vi "Get Signal.vi"(8 "Error in":errorcluster, 10 "Signal Name":string, 11 "CAN Frame in":refnum<class "CAN Frame.lvclass">) -> (0 "error out":errorcluster, 2 "Value":variant, 3 "CAN Frame out":refnum<class "CAN Frame.lvclass">)   [LabVIEW 2023, in "CAN Frame.lvclass"]
uses:
  CAN Frame.lvclass
  CAN Frame.lvclass/CAN Frame.ctl
  CAN Signal/CAN Signal.lvclass/CAN Signal.ctl
  CAN Signal/Get Start Bit.vi
  CAN Signal/Get Bit Length.vi
  CAN Signal/Get Data Type.vi
  CAN Signal/Get Scale.vi
  CAN Signal/Get Offset.vi
  CAN Signal/CAN Signal.lvclass
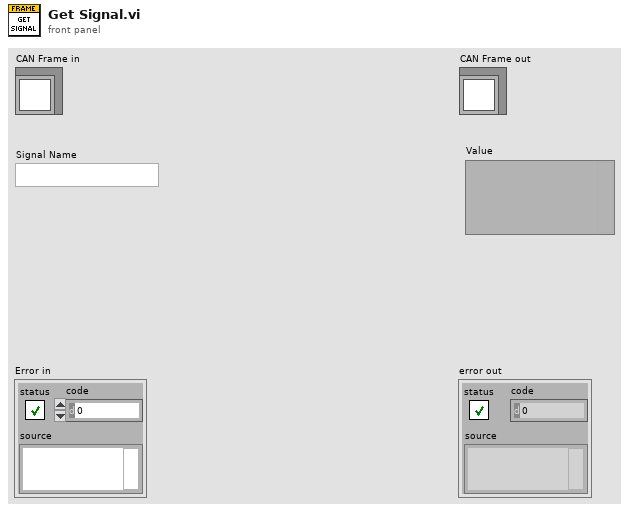
[diagram p1: front panel]
types:
  T1 = enum16{"Signed", "Unsigned", "IEEE Float", "Byte Array"}
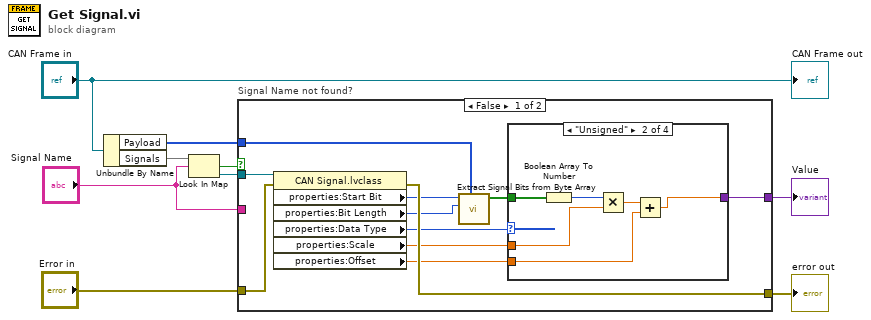
[diagram p0: block diagram]
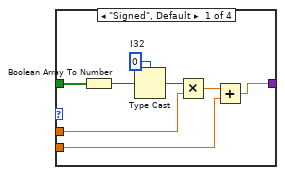
[diagram p2: hidden frame]
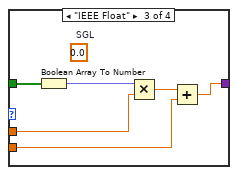
[diagram p3: hidden frame]
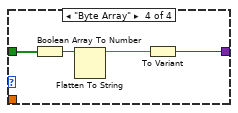
[diagram p4: hidden frame]
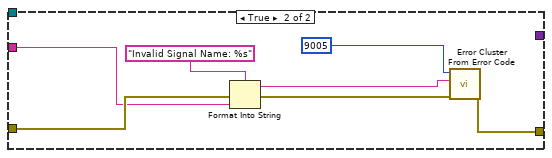
[diagram p5: hidden frame]
diagram:
  n1 = Unbundle By Name("CAN Frame in") -> ("Payload"=w2:u8[], "Signals"=w8:map{string, refnum<class "CAN Signal.lvclass">})
  n2 = Look In Map(map=w8, key="Signal Name") -> (key not found?=w5:bool, value=w6:refnum<class "CAN Signal.lvclass">)  [unwired: 1 in]
  n3 = case "Signal Name not found?" shown="False" w5 {
    tunnel: "Error in" -> [w20 w51]
    tunnel: w6 -> [w19 _]
    tunnel: "Signal Name" -> [_ w46]
    tunnel: [w18 w45] -> w3
    tunnel: w2 -> [w17 _]
    tunnel: [w13 _] -> w1
    frame False {
      n4 = property class="CAN Signal.lvclass"(reference=w19, error in=w20) -> (error out=w18:errorcluster, "properties:Start Bit"=w16:u32, "properties:Bit Length"=w15:u32, "properties:Data Type"=w14:T1, "properties:Scale"=w12:dbl, "properties:Offset"=w11:dbl)  [unwired: 1 out]
      n5 = call "Extract Signal Bits from Byte Array.vi"("Payload"=w17, "Bit Length"=w15, "Start Bit"=w16) -> ("Signal Bits"=w10:bool[])  [unwired: 8 in]
      n6 = case shown="\"Unsigned\"" w14 {
        tunnel: [w24 w31 w39 w43] -> w13
        tunnel: w12 -> [w25 w34 w40 _]
        tunnel: w11 -> [w23 w32 w38 _]
        tunnel: w10 -> [w21 w29 w37 w41]
        frame "Signed", Default {
          w27 = 0  # I32
          n7 = Boolean Array To Number(Boolean array=w21) -> (number=w22:u32)
          n8 = Type Cast(type=w27, x=w22) -> (*(type *) &x=w28:i32)
          n9 = Multiply(x=w28, y=w25) -> (x*y=w26:dbl)
          n10 = Add(x=w26, y=w23) -> (x+y=w24:dbl)
        }
        frame "Unsigned" {
          n11 = Boolean Array To Number(Boolean array=w29) -> (number=w30:u32)
          n12 = Multiply(x=w30, y=w34) -> (x*y=w33:dbl)
          n13 = Add(x=w33, y=w32) -> (x+y=w31:dbl)
        }
        frame "IEEE Float" {
          (unwired) sgl 0.0  # SGL
          n14 = Boolean Array To Number(Boolean array=w37) -> (number=w35:fxp<+/-,32,16>)
          n15 = Multiply(x=w35, y=w40) -> (x*y=w36:dbl)
          n16 = Add(x=w36, y=w38) -> (x+y=w39:dbl)
        }
        frame "Byte Array" {
          n17 = Boolean Array To Number(Boolean array=w41) -> (number=w42:u32)
          n18 = Flatten To String(anything=w42) -> (data string=w44:string)  [unwired: 3 in, 2 out]
          n19 = To Variant(anything=w44) -> (Variant=w43:variant)
        }
      }
    }
    frame True {
      n20 = Format Into String(format string="Invalid Signal Name: %s", error in=w51, w46) -> (resulting string=w48:string, error out=w49:errorcluster)  [unwired: 1 in]
      n21 = call <vilib>:"Error Cluster From Error Code.vi"("error in (no error)"=w49, "error message (\"\")"=w48, "error code (0)"=9005) -> ("error out"=w45:errorcluster)  [unwired: 6 in]
    }
  }
  "error out" <- w3
  "Value" <- w1
  "CAN Frame out" <- "CAN Frame in"
